vi "Receiver.vi"() -> (0 "Channel 7 position":i32, 1 "Channel 6 position":i32, 2 "Channel 5 position":i32, 3 "Channel 4 position":i32, 4 "Value Channel 0":i32)   [LabVIEW 2016]
doc: "Inputs\n-\n\nOutputs\nPosition for channel 4, 5, 6, 7\nValue channel 0\n\nThis VI reads the signals from the RC receiver, process the data and outputs the position on the switches (channel 4. 5, 6, 7) and the value for channel 0 which corresponds to the horisontal positon of the right joystick."
uses:
  <vilib>/rvi/Emulation/niFpgaGetClockAttributes.vi
  <vilib>/rvi/Emulation/niFpgaSctlEmulationGetInTimedLoop.vi
  <vilib>/rvi/Emulation/niFpgaEmulationReportErrorSimple.vi
  <vilib>/rvi/eio/common/nirviEmuTemplateMethod_errors.vi
  <vilib>/rvi/Emulation/niFpgaCriticalErrorInLSC.vi
  <vilib>/eio/EIONode/EIONode.xnode
panel:
  in  "Sync Pulse Max":u32=15000
  in  "Sync Pulse Min":u32=3500
  out "Value Channel 3":u32
  out "Value Channel 2":u32
  out "Value Channel 1":u32
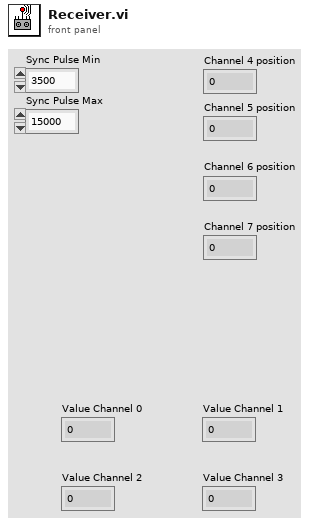
[diagram p1: front panel]
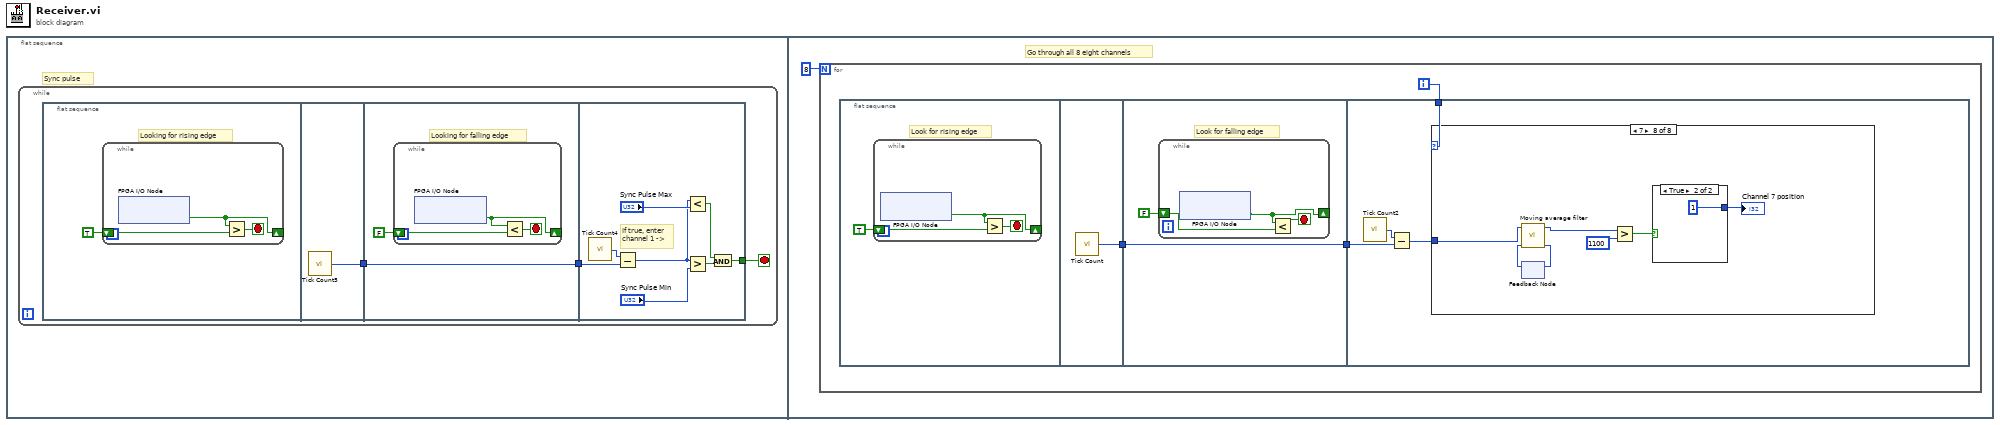
[diagram p0: block diagram]
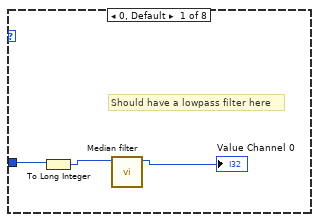
[diagram p2: hidden frame]
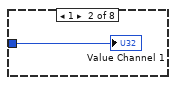
[diagram p3: hidden frame]
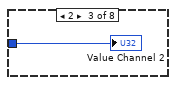
[diagram p4: hidden frame]
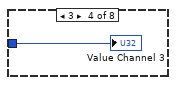
[diagram p5: hidden frame]
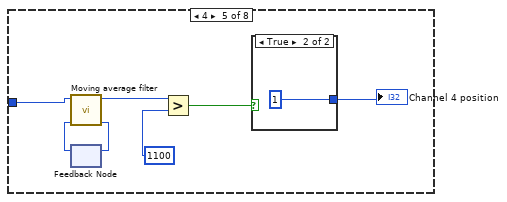
[diagram p6: hidden frame]
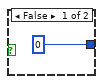
[diagram p7: hidden frame]
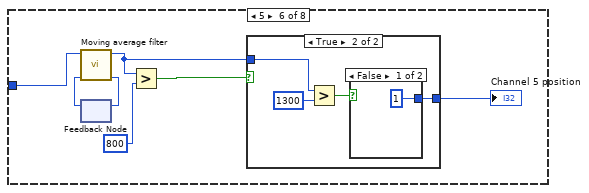
[diagram p8: hidden frame]
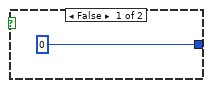
[diagram p9: hidden frame]
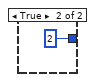
[diagram p10: hidden frame]
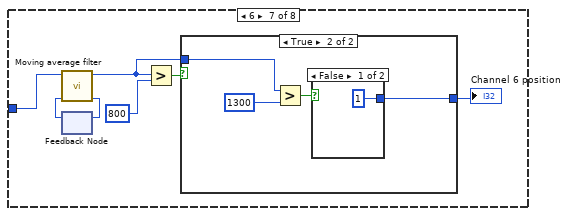
[diagram p11: hidden frame]
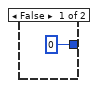
[diagram p12: hidden frame]
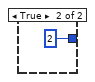
[diagram p13: hidden frame]
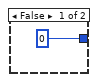
[diagram p14: hidden frame]
diagram:
  n1 = flat-sequence {
    frame #0 {
      # "Sync pulse"
      n2 = while {
        stop <- w1 stop-if-true
        n3 = flat-sequence {
          tunnel: [w8] -> w3
          tunnel: w3 -> [w9]
          tunnel: [w9] -> w2
          tunnel: [w21] -> w1
          tunnel: w2 -> [w16]
          frame #0 {
            # "Looking for rising edge"
            n4 = while {
              shift-right: [w5] -> _
              shift-left: TRUE -> [w6]
              stop <- w7 stop-if-true
              n5 = xnode "FPGA I/O Node"() -> ("DIO/DIO4"=w5:bool)  [unwired: 1 in, 1 out]
              n6 = Greater?(x=w5, y=w6) -> (0:w7:bool)
            }
          }
          frame #1 {
            n7 = call "Tick Count5"() -> ("Tick Count(uSec)"=w8:u32)
          }
          frame #2 {
            # "Looking for falling edge"
            n8 = while {
              shift-right: [w11] -> _
              shift-left: FALSE -> [w12]
              stop <- w13 stop-if-true
              n9 = xnode "FPGA I/O Node"() -> ("DIO/DIO4"=w11:bool)  [unwired: 1 in, 1 out]
              n10 = Less?(x=w11, y=w12) -> (x < y?=w13:bool)
            }
          }
          frame #3 {
            # "If true, enter \nchannel 1 ->"
            n11 = call "Tick Count4"() -> ("Tick Count(uSec)"=w17:u32)
            n12 = Subtract(x=w17, y=w16) -> (x-y=w14:u32)
            n13 = Less?(x=w14, y="Sync Pulse Max") -> (x < y?=w19:bool)
            n14 = Greater?(x=w14, y="Sync Pulse Min") -> (0:w20:bool)
            n15 = And(x=w19, y=w20) -> (x .and. y?=w21:bool)
          }
        }
      }
    }
    frame #1 {
      # "Go through all 8 eight channels"
      n16 = for {
        N: 8 -> [_]
        i -> [w23]
        n17 = flat-sequence {
          tunnel: [w30] -> w25
          tunnel: [w31] -> w24
          tunnel: w25 -> [w31]
          tunnel: w23 -> [w39]
          tunnel: w24 -> [w37]
          frame #0 {
            # "Look for rising edge"
            n18 = while {
              shift-right: [w27] -> _
              shift-left: TRUE -> [w28]
              stop <- w29 stop-if-true
              n19 = xnode "FPGA I/O Node"() -> ("DIO/DIO4"=w27:bool)  [unwired: 1 in, 1 out]
              n20 = Greater?(x=w27, y=w28) -> (0:w29:bool)
            }
          }
          frame #1 {
            n21 = call "Tick Count"() -> ("Tick Count(uSec)"=w30:u32)
          }
          frame #2 {
            # "Look for falling edge"
            n22 = while {
              shift-right: [w33] -> _
              shift-left: FALSE -> [w34]
              stop <- w35 stop-if-true
              n23 = xnode "FPGA I/O Node"() -> ("DIO/DIO4"=w33:bool)  [unwired: 1 in, 1 out]
              n24 = Less?(x=w33, y=w34) -> (x < y?=w35:bool)
            }
          }
          frame #3 {
            n25 = call "Tick Count2"() -> ("Tick Count(uSec)"=w38:u32)
            n26 = Subtract(x=w38, y=w37) -> (x-y=w36:u32)
            n27 = case shown="7" w39 {
              tunnel: w36 -> [w41 w43 w44 w45 w48 w56 w70 w85]
              frame 0, Default {
                # "Should have a lowpass filter here"
                n28 = To Long Integer(number=w41) -> (32bit integer=w40:i32)
                n29 = call "Median filter.vi"("Rawdata"=w40) -> ("Filtered element"=→"Value Channel 0":i32)  [unwired: 10 in]
              }
              frame 1 {
                "Value Channel 1" <- w43
              }
              frame 2 {
                "Value Channel 2" <- w44
              }
              frame 3 {
                "Value Channel 3" <- w45
              }
              frame 4 {
                n30 = feedback #1() -> (w47:i32)  [unwired: 1 in]
                n31 = call "Moving average filter.vi"("x"=w47, "Input"=w48) -> ("xdot"=w46:i32, "Mean"=w49:i32)  [unwired: 8 in]
                n32 = feedback-in #1(w46) -> ()
                n33 = Greater?(x=w49, y=1100) -> (0:w51:bool)
                n34 = case shown="True" w51 {
                  tunnel: [0 1] -> w50
                  frame False {
                  }
                  frame True {
                  }
                }
                "Channel 4 position" <- w50
              }
              frame 5 {
                n35 = feedback #2() -> (w59:i32)  [unwired: 1 in]
                n36 = call "Moving average filter.vi"("x"=w59, "Input"=w56) -> ("xdot"=w58:i32, "Mean"=w57:i32)  [unwired: 8 in]
                n37 = feedback-in #2(w58) -> ()
                n38 = Greater?(x=w57, y=800) -> (0:w61:bool)
                n39 = case shown="True" w61 {
                  tunnel: w57 -> [_ w65]
                  tunnel: [0 w63] -> w60
                  frame False {
                  }
                  frame True {
                    n40 = Greater?(x=w65, y=1300) -> (0:w66:bool)
                    n41 = case shown="False" w66 {
                      tunnel: [1 2] -> w63
                      frame False {
                      }
                      frame True {
                      }
                    }
                  }
                }
                "Channel 5 position" <- w60
              }
              frame 6 {
                n42 = feedback #3() -> (w72:i32)  [unwired: 1 in]
                n43 = call "Moving average filter.vi"("x"=w72, "Input"=w70) -> ("xdot"=w71:i32, "Mean"=w69:i32)  [unwired: 8 in]
                n44 = feedback-in #3(w71) -> ()
                n45 = Greater?(x=w69, y=800) -> (0:w74:bool)
                n46 = case shown="True" w74 {
                  tunnel: w69 -> [_ w79]
                  tunnel: [0 w78] -> w75
                  frame False {
                  }
                  frame True {
                    n47 = Greater?(x=w79, y=1300) -> (0:w80:bool)
                    n48 = case shown="False" w80 {
                      tunnel: [1 2] -> w78
                      frame False {
                      }
                      frame True {
                      }
                    }
                  }
                }
                "Channel 6 position" <- w75
              }
              frame 7 {
                n49 = feedback #4() -> (w84:i32)  [unwired: 1 in]
                n50 = call "Moving average filter.vi"("x"=w84, "Input"=w85) -> ("xdot"=w83:i32, "Mean"=w86:i32)  [unwired: 8 in]
                n51 = feedback-in #4(w83) -> ()
                n52 = Greater?(x=w86, y=1100) -> (0:w89:bool)
                n53 = case shown="True" w89 {
                  tunnel: [0 1] -> w87
                  frame False {
                  }
                  frame True {
                  }
                }
                "Channel 7 position" <- w87
              }
            }
          }
        }
      }
    }
  }
